vi "Project.Close.vi"(10 "Project File Path":path, 11 "Gateway IP Address (\"\": localhost)":string) -> (0 "error out":errorcluster)   [LabVIEW 2013, in "MiscHelperVIs.lvlib"]
uses:
  MiscHelperVIs.lvlib
  <vilib>/NI Veristand/Execution/Project/NI_VS Project ExecutionAPI.lvlib
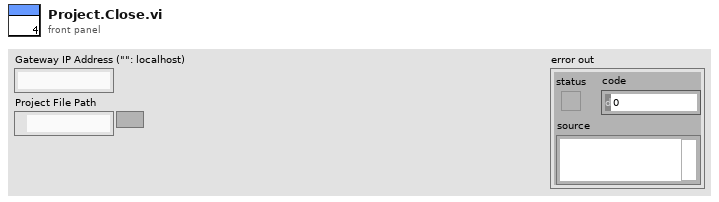
[diagram p1: front panel]
types:
  T1 = typedef "NI_VS Project ExecutionAPI.lvlib/Project Ref.ctl" = refnum<k24>
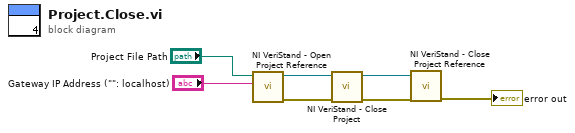
[diagram p0: block diagram]
diagram:
  n1 = call <vilib>:"NI VeriStand - Open Project Reference.vi"("Gateway IP Address (\"\": localhost)"="Gateway IP Address (\"\": localhost)", "Project File Path"="Project File Path") -> ("error out"=w5:errorcluster, "Project Ref"=w4:T1)  [unwired: 8 in]
  n2 = call <vilib>:"NI VeriStand - Close Project.vi"("error in (no error)"=w5, "Project Ref in"=w4) -> ("error out"=w2:errorcluster, "Project Ref out"=w3:T1)  [unwired: 8 in]
  n3 = call <vilib>:"NI VeriStand - Close Project Reference.vi"("error in (no error)"=w2, "Project Ref"=w3) -> ("error out"=→"error out":errorcluster)  [unwired: 9 in]
